vi "Mass Flow Sensor.vi"() -> ()   [LabVIEW 2019]
uses:
  <vilib>/express/express shared/transition.llb/Dynamic To Waveform Array.vi
  <vilib>/express/express arith-compare/Formula/Block/exnFormulaBlock how many pts in the wave.vi
  <vilib>/express/express shared/ex_Modify Signal Name.vi
  <vilib>/express/express shared/transition.llb/Waveform Array To Dynamic.vi
  <vilib>/express/express arith-compare/Formula/XNode/ExpressFormulaBlockNode.xnode
panel:
  out "Voltage 1":dbl format="%#.2g"
  out "Average CFM 1":dbl format="%.1g"
  out "CFM 1":dbl format="%.2g"
  out "Average CFM 2":dbl format="%.1g"
  out "CFM 2":dbl format="%.2g"
  out "Voltage 2":dbl format="%#.2g"
  out "Average CFM 3":dbl format="%.1g"
  out "CFM 3":dbl format="%.2g"
  out "Voltage 3":dbl format="%.2g"
  in  "stop":bool
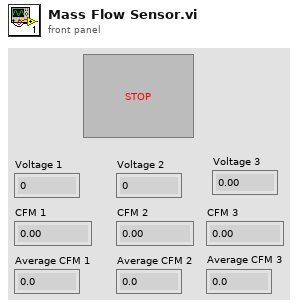
[diagram p1: front panel]
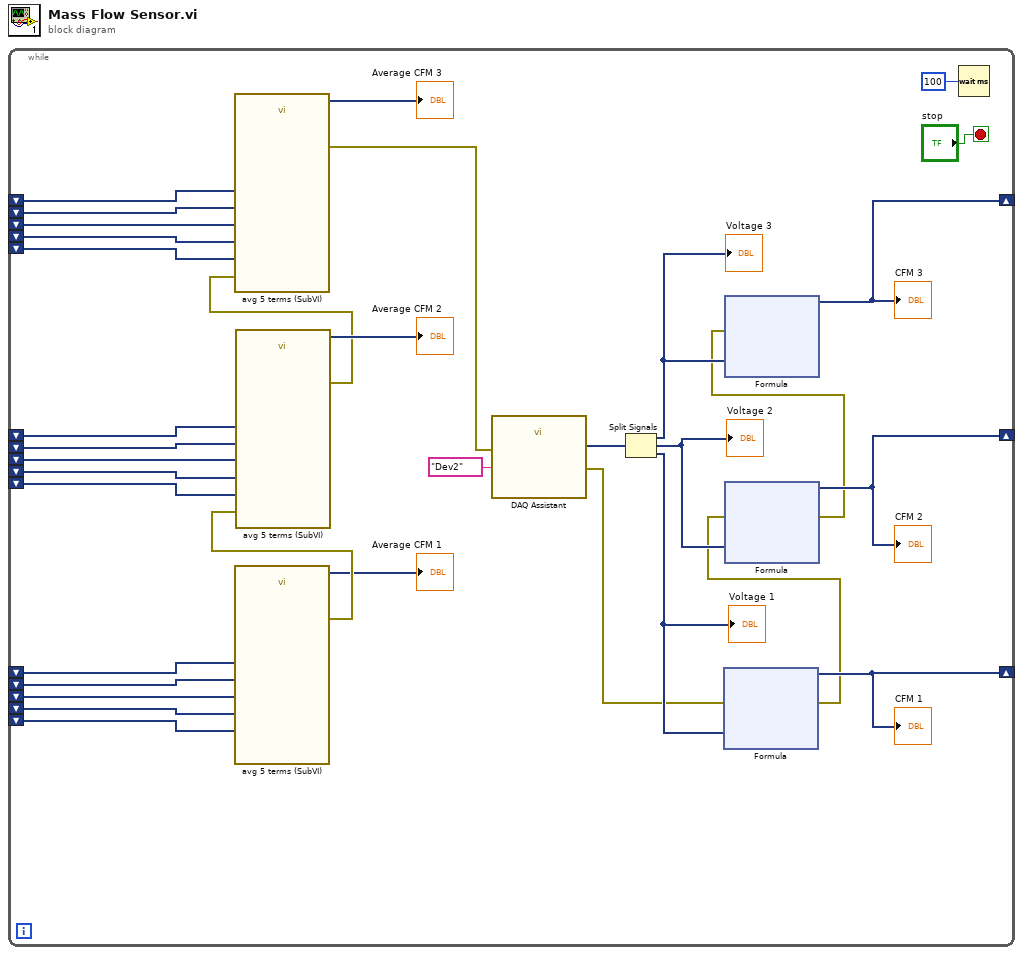
[diagram p0: block diagram]
diagram:
  n1 = while {
    shift-right: [w22] -> _
    shift-left: _ -> [w6]
    shift-left: _ -> [w11]
    shift-left: _ -> [w8]
    shift-right: [w25] -> _
    shift-left: _ -> [w30]
    shift-left: _ -> [w32]
    shift-left: _ -> [w31]
    shift-left: _ -> [w7]
    shift-left: _ -> [w12]
    shift-left: _ -> [w28]
    shift-left: _ -> [w27]
    shift-right: [w24] -> _
    shift-left: _ -> [w13]
    shift-left: _ -> [w14]
    shift-left: _ -> [w15]
    shift-left: _ -> [w16]
    shift-left: _ -> [w17]
    stop <- "stop" stop-if-true
    n2 = call "avg 5 terms (SubVI).vi"("Result"=w17, "Result 3"=w13, "Result 4"=w16, "Result 5"=w15, "Result 2"=w14) -> ("error out"=w19:errorcluster, "Dynamic Data"=→"Average CFM 1":dynamicdata)  [unwired: 5 in]
    n3 = call "avg 5 terms (SubVI).vi"("Result"=w27, "Result 3"=w30, "error in (no error)"=w19, "Result 4"=w31, "Result 5"=w32, "Result 2"=w28) -> ("error out"=w10:errorcluster, "Dynamic Data"=→"Average CFM 2":dynamicdata)  [unwired: 4 in]
    n4 = call "avg 5 terms (SubVI).vi"("Result"=w12, "Result 3"=w6, "error in (no error)"=w10, "Result 4"=w11, "Result 5"=w8, "Result 2"=w7) -> ("error out"=w9:errorcluster, "Dynamic Data"=→"Average CFM 3":dynamicdata)  [unwired: 4 in]
    n5 = call "DAQ Assistant"("error in"=w9, "device name"=tag "Dev2") -> ("data"=w29:dynamicdata, "error out"=w4:errorcluster)  [unwired: 15 in, 1 out]
    n6 = Split Signals(w29) -> (w20:dynamicdata, w21:dynamicdata, w23:dynamicdata)  [unwired: 3 in]
    "Voltage 3" <- w20
    "Voltage 2" <- w21
    "Voltage 1" <- w23
    n7 = xnode "Formula"("X1"=w23, "error in (no error)"=w4) -> ("Result"=w24:dynamicdata, "error out"=w3:errorcluster)
    "CFM 1" <- w24
    n8 = xnode "Formula"("X1"=w21, "error in (no error)"=w3) -> ("Result"=w25:dynamicdata, "error out"=w2:errorcluster)
    "CFM 2" <- w25
    n9 = xnode "Formula"("X1"=w20, "error in (no error)"=w2) -> ("Result"=w22:dynamicdata)  [unwired: 1 out]
    "CFM 3" <- w22
    n10 = Wait (ms)(milliseconds to wait=u32 100 ("millisecond timer value")) -> ()  [unwired: 1 out]
  }
